vi "Configure Serial Bus (M1553 - Autosetup).vi"(0 "VISA resource name":refnum<visa-resource-name>, 5 "Serial Bus Name (1: Serial Bus 1)":i32(ring)=1 items=["Serial Bus 1"=1, "Serial Bus 2"=2], 11 "error in (no error)":errorcluster) -> (4 "VISA resource name out":refnum<visa-resource-name>, 15 "error out":errorcluster)   [LabVIEW 2016, in "Agilent 2000 3000 X-Series.lvlib"]
doc: "Sets these options for decoding and triggering on MIL- STD- 1553 signals automatically:\n\nHigh/Low Trigger Thresholds: to a voltage value equal to 1/3 division\nbased on the source channel's current V/div setting.\n\nNoise Reject: Off.\n\nProbe Attenuation: 10.0.\n\nSerial Decode: On.\n\nTrigger: the specified serial bus (n of SBUS<n>)."
uses:
  Agilent 2000 3000 X-Series.lvlib
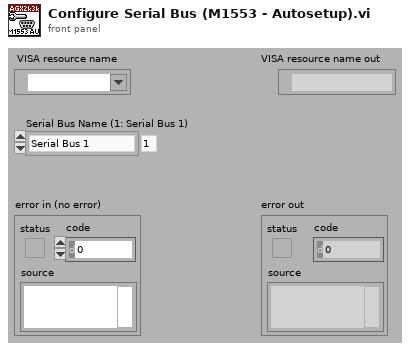
[diagram p1: front panel]
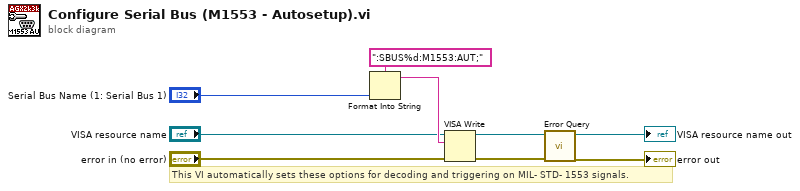
[diagram p0: block diagram]
diagram:
  # "This VI automatically sets these options for decoding and triggering on MIL- STD- 1553 signals."
  n1 = Format Into String(format string=":SBUS%d:M1553:AUT;", "Serial Bus Name (1: Serial Bus 1)") -> (resulting string=w7:string)  [unwired: 2 in, 1 out]
  n2 = VISA Write(VISA resource name="VISA resource name", write buffer=w7, error in (no error)="error in (no error)") -> (VISA resource name out=w4:refnum<visa-resource-name>, error out=w3:errorcluster)  [unwired: 1 out]
  n3 = call "Error Query.vi"("error in (no error)"=w3, "VISA resource name"=w4) -> ("error out"=→"error out":errorcluster, "VISA resource name out"=→"VISA resource name out":refnum<visa-resource-name>)  [unwired: 8 out]
